vi "Read Vacuum Channels.vi"(8 "error in (no error)":errorcluster, 11 "GH2 in":refnum<class "GH2.lvclass">) -> (0 "error out":errorcluster, 2 "Vacuum Channels":bool[](array[boolean]), 3 "GH2 out":refnum<class "GH2.lvclass">)   [LabVIEW 2026, in "GH2.lvclass"]
uses:
  GH2.lvclass
  GH2.lvclass/GH2.ctl
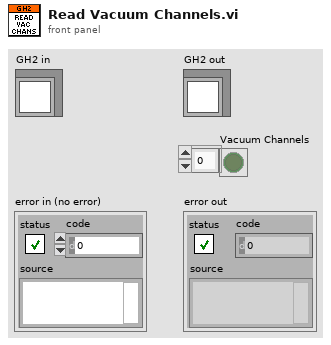
[diagram p1: front panel]
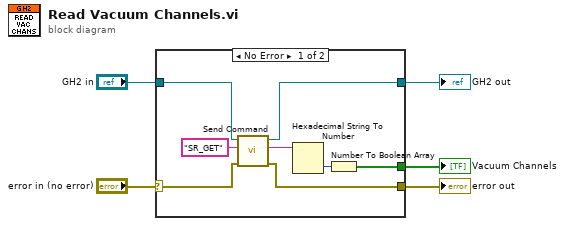
[diagram p0: block diagram]
diagram:
  n1 = case shown="No Error" "error in (no error)" {
    selector: "error in (no error)" -> [w12 w15]
    tunnel: [w9 w15] -> w4
    tunnel: [w10 w14] -> w2
    tunnel: "GH2 in" -> [w11 w14]
    tunnel: [w6 _] -> w1
    frame No Error {
      n2 = call "Send Command.vi"("error in (no error)"=w12, "command"="SR_GET", "GH2 in"=w11) -> ("error out"=w9:errorcluster, "response"=w7:string, "GH2 out"=w10:refnum<class "GH2.lvclass">)  [unwired: 6 in]
      n3 = Hexadecimal String To Number(string=w7) -> (number=w8:u32)  [unwired: 2 in, 1 out]
      n4 = Number To Boolean Array(number=w8) -> (Boolean array=w6:bool[])
    }
    frame Error {
    }
  }
  "error out" <- w4
  "GH2 out" <- w2
  "Vacuum Channels" <- w1
